vi "main.vi"() -> ()   [LabVIEW 2023]
panel:
  out "Version":string
  in  "Error IN":errorcluster
  out "error IO":errorcluster
  in  "stop":bool
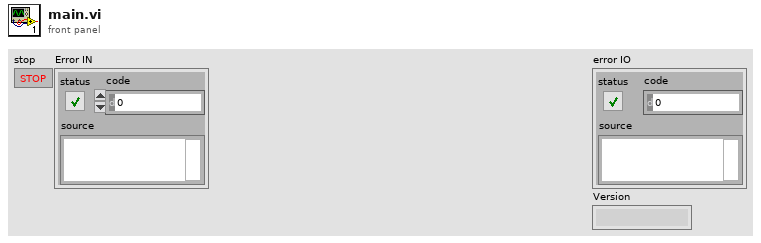
[diagram p1: front panel]
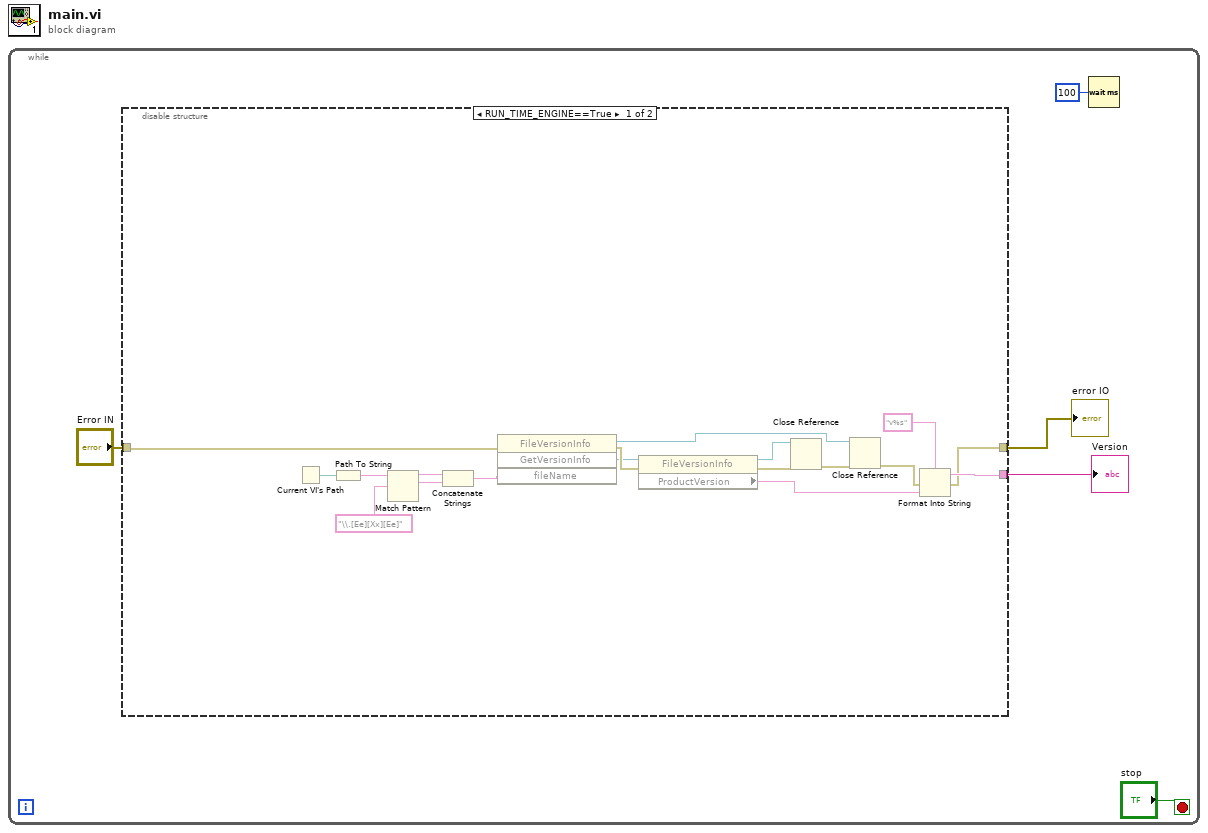
[diagram p0: block diagram]
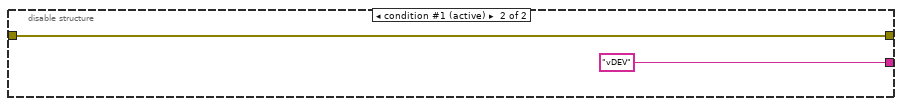
[diagram p2: hidden frame]
diagram:
  n1 = while {
    stop <- "stop" stop-if-true
    n2 = disable-structure shown="RUN_TIME_ENGINE==True" {
      disable-tunnel: "Error IN" -> [w12 w25]
      disable-tunnel: [w22 w25] -> w3
      disable-tunnel: [w23 "vDEV" ("Version")] -> w1
      frame condition #0 {
        n3 = Current VI's Path() -> (path=w11:path)
        n4 = Path To String(path=w11) -> (string=w7:string)
        n5 = Match Pattern(string=w7, regular expression="\\.[Ee][Xx][Ee]") -> (before substring=w8:string, match substring=w9:string)  [unwired: 1 in, 2 out]
        n6 = Concatenate Strings(w8, w9) -> (w6:string)
        n7 = invoke class="FileVersionInfo" method="GetVersionInfo"(error in=w12, "fileName"=w6) -> (reference out=w20:refnum<k24>, error out=w16:errorcluster, "GetVersionInfo"=w15:refnum<k24>)  [unwired: 2 in, 1 out]
        n8 = property class="FileVersionInfo"(reference=w15, error in=w16) -> (reference out=w19:refnum<k24>, error out=w17:errorcluster, "ProductVersion"=w13:string)
        n9 = Close Reference(reference=w19, error in (no error)=w17) -> (error out=w18:errorcluster)
        n10 = Close Reference(reference=w20, error in (no error)=w18) -> (error out=w14:errorcluster)
        n11 = Format Into String(format string="v%s", error in=w14, w13) -> (resulting string=w23:string, error out=w22:errorcluster)  [unwired: 1 in]
      }
      frame condition #1 (active) {
      }
    }
    "error IO" <- w3
    "Version" <- w1
    n12 = Wait (ms)(milliseconds to wait=u32 100) -> ()  [unwired: 1 out]
  }
